vi "completeImage.vi"(6 "Times In":u32[](array[numeric]), 8 "Numeric":i32, 9 "file (use dialog)":path=path "C:/Users/Chuck Randy/Desktop/asdf.jpg", 10 "Array":u16[](array[numeric]), 11 "InputImages":T1(array[cluster])) -> (0 "Numeric 2":i32, 2 "Array 2":u16[](array[numeric]), 3 "OutputImages":T1(array[cluster]), 4 "Times Out":u32[](array[numeric]))   [LabVIEW 2014]
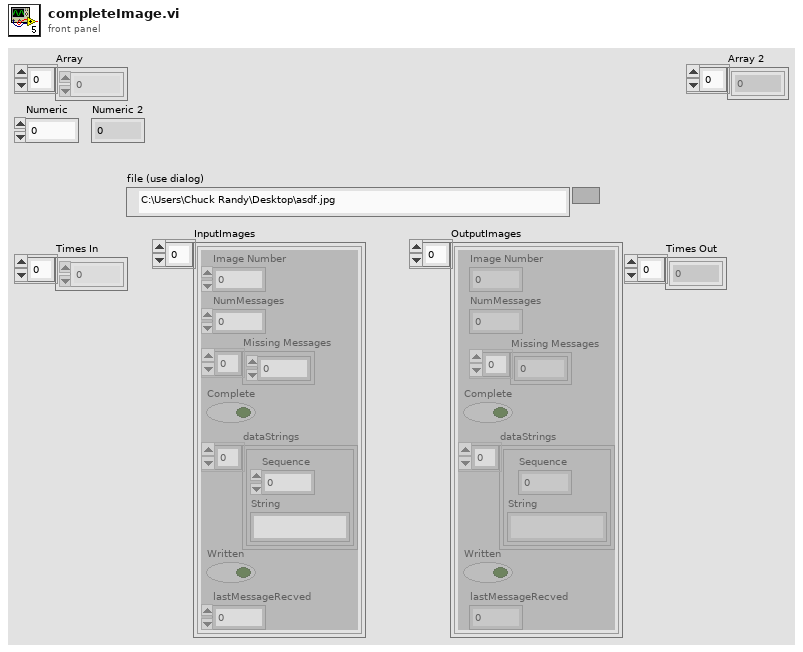
[diagram p1: front panel]
types:
  T1 = cluster{"Image Number":u16, "NumMessages":u16, "Missing Messages":u16[], "Complete":bool, "dataStrings":cluster{"Sequence":u16, "String":string}[], "Written":bool, "lastMessageRecved":u32}[]
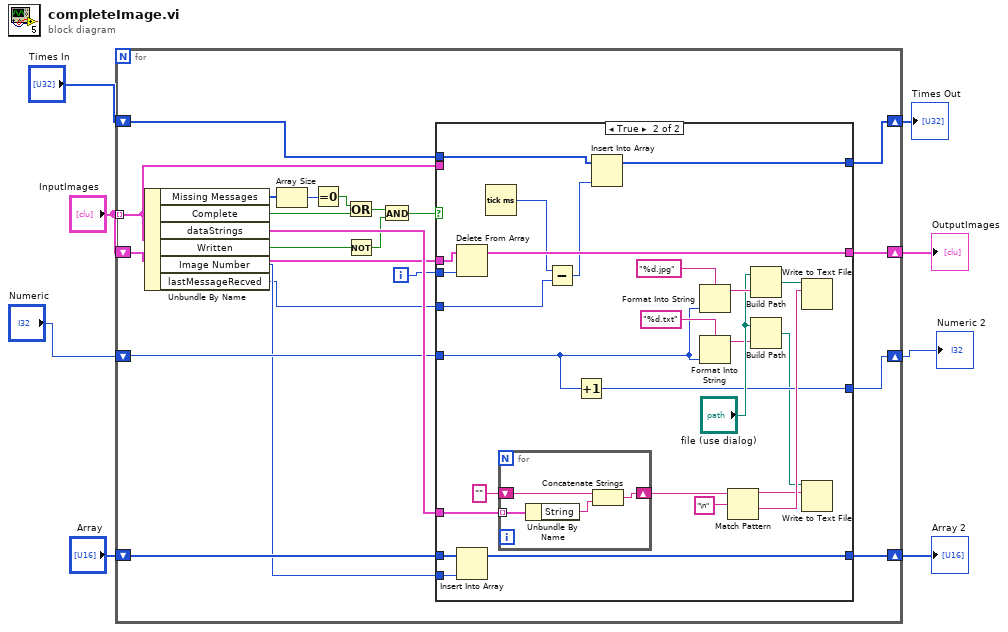
[diagram p0: block diagram]
diagram:
  n1 = for {
    tunnel: "InputImages" -> [w28] mode=indexing
    shift-right: [w27] -> w8
    shift-left: "InputImages" -> [w26]
    shift-right: [w21] -> w6
    shift-left: "Array" -> [w20]
    shift-right: [w13] -> w3
    shift-left: "Numeric" -> [w14]
    shift-right: [w9] -> w1
    shift-left: "Times In" -> [w10]
    i -> [w19]
    n2 = Unbundle By Name(w28) -> ("Missing Messages"=w18:u16[], "Complete"=w24:bool, "dataStrings"=w29:cluster{"Sequence":u16, "String":string}[], "Written"=w25:bool, "Image Number"=w12:u16, "lastMessageRecved"=w11:u32)
    n3 = Array Size(array=w18) -> (size(s)=w17:i32)
    n4 = Equal To 0?(x=w17) -> (x = 0?=w15:bool)
    n5 = Or(x=w15, y=w24) -> (x .or. y?=w16:bool)
    n6 = Not(x=w25) -> (.not. x?=w23:bool)
    n7 = And(x=w16, y=w23) -> (x .and. y?=w22:bool)
    n8 = case shown="True" w22 {
      tunnel: w29 -> [_ w48]
      tunnel: w14 -> [w31 w42]
      tunnel: w28 -> [_ _]
      tunnel: [w32 w43] -> w27
      tunnel: w26 -> [w32 w45]
      tunnel: [w33 w47] -> w21
      tunnel: w20 -> [w33 w46]
      tunnel: w19 -> [_ w44]
      tunnel: [w31 w41] -> w13
      tunnel: w12 -> [_ w40]
      tunnel: w11 -> [_ w39]
      tunnel: w10 -> [w30 w37]
      tunnel: [w30 w35] -> w9
      frame False {
      }
      frame True {
        n9 = Delete From Array(array=w45, index=w44) -> (array with subset deleted=w43:T1)  [unwired: 1 in, 1 out]
        n10 = Insert Into Array(array=w46, new element=w40) -> (w47:u16[])  [unwired: 1 in]
        n11 = Tick Count (ms)() -> (millisecond timer value=w38:u32)
        n12 = for {
          tunnel: w48 -> [w61] mode=indexing
          shift-right: [w63] -> w58
          shift-left: "" -> [w62]
          n13 = Unbundle By Name(w61) -> ("String"=w60:string)
          n14 = Concatenate Strings(w62, w60) -> (w63:string)
        }
        n15 = Subtract(x=w38, y=w39) -> (x-y=w36:u32)
        n16 = Increment(x=w42) -> (x+1=w41:i32)
        n17 = Insert Into Array(array=w37, new element=w36) -> (w35:u32[])  [unwired: 1 in]
        n18 = Format Into String(format string="%d.jpg", w42) -> (resulting string=w53:string)  [unwired: 2 in, 1 out]
        n19 = Format Into String(format string="%d.txt", w42) -> (resulting string=w50:string)  [unwired: 2 in, 1 out]
        n20 = Match Pattern(string=w58, regular expression="\n") -> (before substring=w49:string, after substring=w56:string)  [unwired: 1 in, 2 out]
        n21 = Build Path(base path="file (use dialog)", name or relative path=w53) -> (appended path=w52:path)
        n22 = Build Path(base path="file (use dialog)", name or relative path=w50) -> (appended path=w34:path)
        n23 = Write to Text File(file (use dialog)=w52, text=w56) -> ()  [unwired: 2 in, 3 out]
        n24 = Write to Text File(file (use dialog)=w34, text=w49) -> ()  [unwired: 2 in, 3 out]
      }
    }
  }
  "OutputImages" <- w8
  "Array 2" <- w6
  "Numeric 2" <- w3
  "Times Out" <- w1
